vi "LV diagram nodes.vi"(8 "error in (no error)":errorcluster, 11 "diagrams in":T1(array[cluster])) -> (2 "diagram desc.":string, 3 "diagrams out":T1(array[cluster]))   [LabVIEW 2012]
panel:
  out "error out":errorcluster
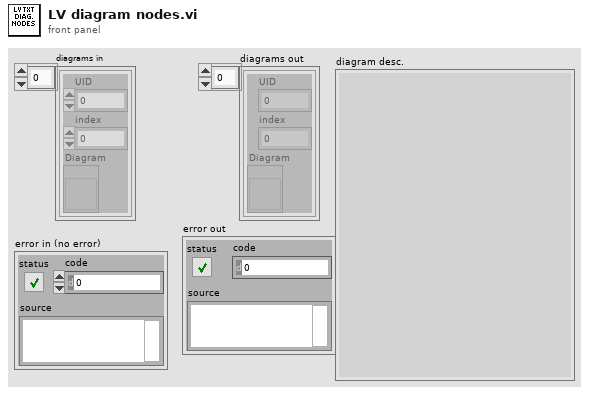
[diagram p1: front panel]
types:
  T1 = cluster{"UID":i32, "index":i32, "Diagram":refnum<vi>}[]
  T2 = cluster{"UID":i32, "index":i32, "Diagram":refnum<vi>}
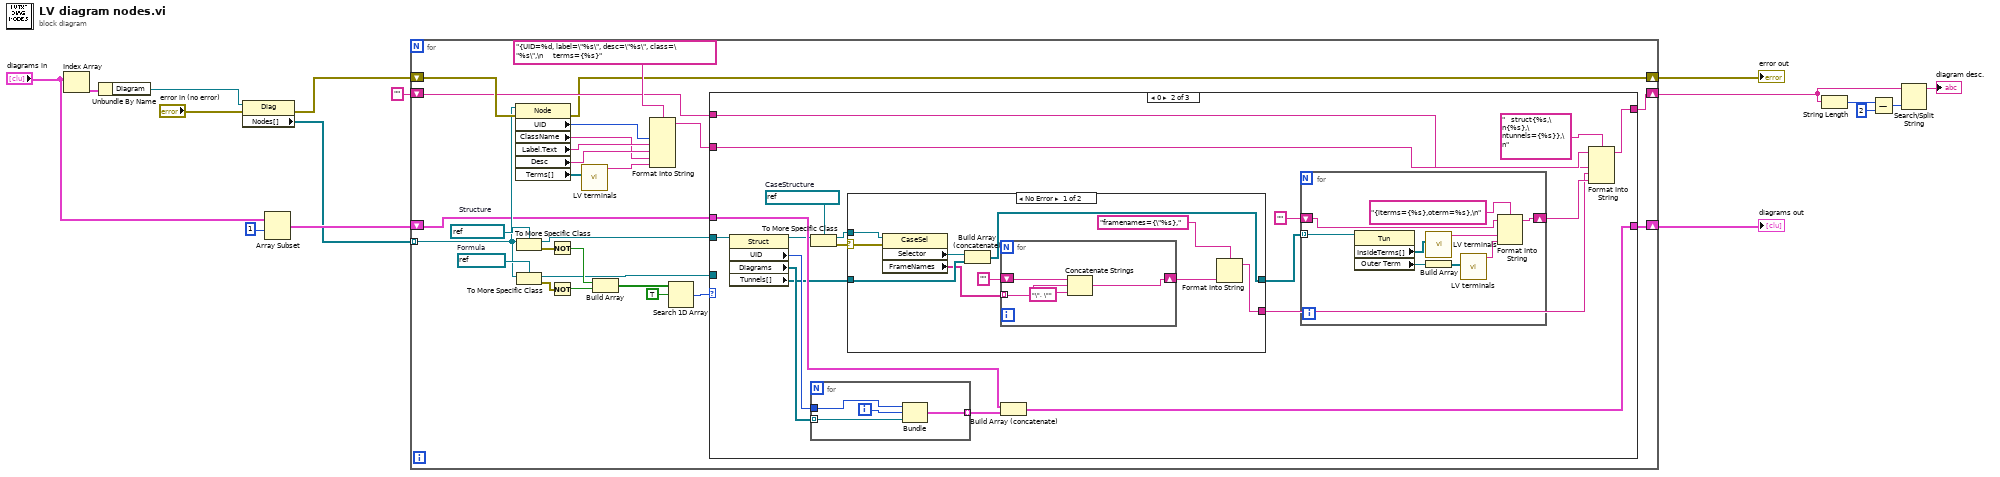
[diagram p0: block diagram]
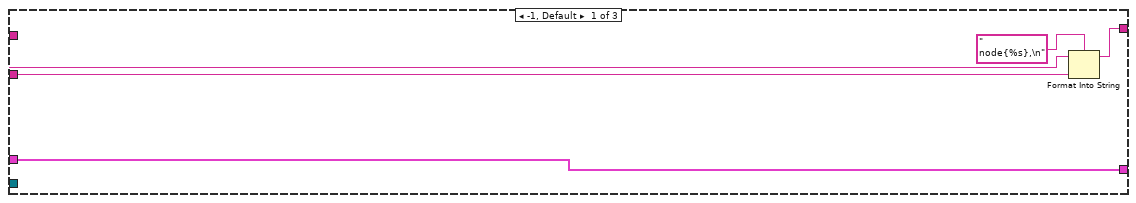
[diagram p2: hidden frame]
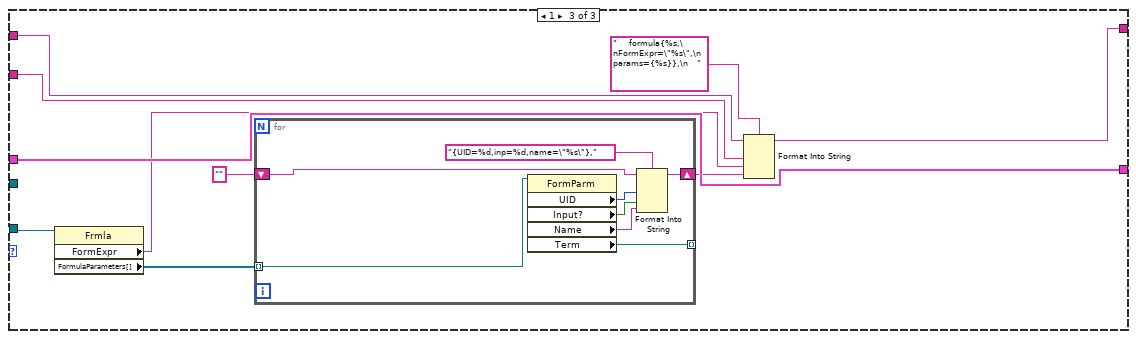
[diagram p4: hidden frame]
diagram:
  n1 = Index Array(array="diagrams in") -> (element=w16:T2)  [unwired: 1 in]
  n2 = Unbundle By Name(w16) -> ("Diagram"=w14:refnum<vi>)
  n3 = property class="Diag"(reference=w14, error in="error in (no error)") -> (error out=w7:errorcluster, "Nodes[]"=w6:refnum<vi>[])  [unwired: 1 out]
  n4 = Array Subset(array="diagrams in", index=1) -> (w10:T1)  [unwired: 1 in]
  n5 = for {
    tunnel: w6 -> [w35] mode=indexing
    shift-right: [w18] -> w5
    shift-left: "" -> [w19]
    shift-right: [w25] -> w11
    shift-left: w10 -> [w26]
    shift-right: [w17] -> w1
    shift-left: w7 -> [w38]
    w36 = refnum<vi> refnum  # Formula
    w37 = refnum<vi> refnum  # Structure
    n6 = property class="Node"(reference=w35, error in=w38) -> (error out=w17:errorcluster, "UID"=w42:i32, "ClassName"=w21:string, "Label.Text"=w40:string, "Desc"=w39:string, "Terms[]"=w23:refnum<vi>[])  [unwired: 1 out]
    n7 = To More Specific Class(target class=w37, reference=w35) -> (specific class reference=w27:refnum<vi>, error out=w34:errorcluster)  [unwired: 1 in]
    n8 = To More Specific Class(target class=w36, reference=w35) -> (specific class reference=w24:refnum<vi>, error out=w33:errorcluster)  [unwired: 1 in]
    n9 = Not(x=w34) -> (.not. x?=w32:bool)
    n10 = Not(x=w33) -> (.not. x?=w31:bool)
    n11 = call "LV terminals.vi"("Terms[]"=w23) -> ("String out"=w22:string)  [unwired: 9 in, 1 out]
    n12 = Build Array(w32, w31) -> (w30:bool[])
    n13 = Format Into String(format string="{UID=%d, label=\"%s\", desc=\"%s\", class=\"%s\",\n     terms={%s}", w42, w40, w39, w21, w22) -> (resulting string=w20:string)  [unwired: 2 in, 1 out]
    n14 = Search 1D Array(1D array=w30, element=TRUE) -> (index of element=w28:i32)  [unwired: 1 in]
    n15 = case shown="0" w28 {
      tunnel: w27 -> [_ w64 _]
      tunnel: w26 -> [w47 w62 w104]
      tunnel: [w47 w61 w104] -> w25
      tunnel: w24 -> [_ _ w103]
      tunnel: w20 -> [w45 w49 w96]
      tunnel: w19 -> [w44 w58 w95]
      tunnel: [w43 w56 w97] -> w18
      frame -1, Default {
        n16 = Format Into String(format string="   node{%s},\n" ("string"), initial string=w44, w45) -> (resulting string=w43:string)  [unwired: 1 in, 1 out]
      }
      frame 0 {
        w55 = refnum<vi> refnum  # CaseStructure
        n17 = property class="Struct"(reference=w64) -> (reference out=w52:refnum<vi>, "UID"=w66:i32, "Diagrams"=w65:refnum<vi>[], "Tunnels[]"=w51:refnum<vi>[])  [unwired: 1 in, 1 out]
        n18 = To More Specific Class(target class=w55, reference=w52) -> (specific class reference=w54:refnum<vi>, error out=w53:errorcluster)  [unwired: 1 in]
        n19 = for {
          tunnel: w65 -> [w94] mode=indexing
          tunnel: w66 -> [w92]
          tunnel: [w93] -> w63 mode=indexing
          i -> [w91]
          n20 = Bundle("UID"=w92, w91, w94) -> (w93:cluster{"UID":i32, i32, refnum<vi>})  [unwired: 1 in]
        }
        n21 = case shown="No Error" w53 {
          selector: w53 -> [w75 _]
          tunnel: w54 -> [w76 _]
          tunnel: w51 -> [w73 w81]
          tunnel: [w72 w81] -> w50
          tunnel: [w69 _] -> w48
          frame No Error {
            n22 = property class="CaseSel"(reference=w76, error in=w75) -> ("Selector"=w74:refnum<vi>, "FrameNames"=w71:string[])  [unwired: 2 out]
            n23 = Build Array (concatenate)(w74, w73) -> (w72:refnum<vi>[])
            n24 = for {
              tunnel: w71 -> [w80] mode=indexing
              shift-right: [w78] -> w67
              shift-left: "" -> [w77]
              n25 = Concatenate Strings(w77, w80, "\", \"" ("string")) -> (w78:string)
            }
            n26 = Format Into String(format string="framenames={\"%s}," ("string"), w67) -> (resulting string=w69:string)  [unwired: 2 in, 1 out]
          }
          frame Error {
          }
        }
        n27 = Build Array (concatenate)(w62, w63) -> (w61:T1)
        n28 = for {
          shift-right: [w85] -> w57
          shift-left: "" -> [w86]
          tunnel: w50 -> [w84] mode=indexing
          n29 = property class="Tun"(reference=w84) -> ("InsideTerms[]"=w90:refnum<vi>[], "Outer Term"=w83:refnum<vi>)  [unwired: 1 in, 2 out]
          n30 = call "LV terminals.vi"("Terms[]"=w90) -> ("String out"=w87:string)  [unwired: 9 in, 1 out]
          n31 = Build Array(w83) -> (w89:refnum<vi>[])
          n32 = call "LV terminals.vi"("Terms[]"=w89) -> ("String out"=w82:string)  [unwired: 9 in, 1 out]
          n33 = Format Into String(format string="{iterms={%s},oterm=%s},\n", initial string=w86, w87, w82) -> (resulting string=w85:string)  [unwired: 1 in, 1 out]
        }
        n34 = Format Into String(format string="   struct{%s,\n{%s},\ntunnels={%s}},\n" ("string"), initial string=w58, w49, w48, w57) -> (resulting string=w56:string)  [unwired: 1 in, 1 out]
      }
      frame 1 {
        n35 = property class="Frmla"(reference=w103) -> ("FormExpr"=w99:string, "FormulaParameters[]"=w102:refnum<vi>[])  [unwired: 1 in, 2 out]
        n36 = for {
          tunnel: w102 -> [w112] mode=indexing
          tunnel: [w111] -> _ mode=indexing
          shift-right: [w107] -> w98
          shift-left: "" -> [w106]
          n37 = property class="FormParm"(reference=w112) -> ("UID"=w110:i32, "Input?"=w109:bool, "Name"=w108:string, "Term"=w111:refnum<vi>)  [unwired: 1 in, 2 out]
          n38 = Format Into String(format string="{UID=%d,inp=%d,name=\"%s\"},", initial string=w106, w110, w109, w108) -> (resulting string=w107:string)  [unwired: 1 in, 1 out]
        }
        n39 = Format Into String(format string="    formula{%s,\nFormExpr=\"%s\",\n    params={%s}},\n   ", initial string=w95, w96, w99, w98) -> (resulting string=w97:string)  [unwired: 1 in, 1 out]
      }
    }
  }
  "diagrams out" <- w11
  "error out" <- w1
  n40 = String Length(string=w5) -> (length=w4:i32)
  n41 = Subtract(x=w4, y=2) -> (x-y=w2:i32)
  n42 = Search/Split String(string=w5, offset (0)=w2) -> (substring before match=→"diagram desc.":string)  [unwired: 1 in, 2 out]
